vi "Close binary videos refs.vi"(8 "error in":errorcluster, 11 "Cam Binary Videos":refnum<file>[](array[refnum])) -> (0 "error out (no error)":errorcluster)   [LabVIEW 2013]
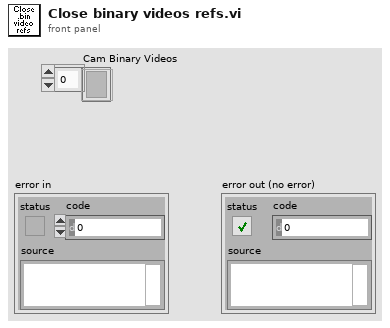
[diagram p1: front panel]
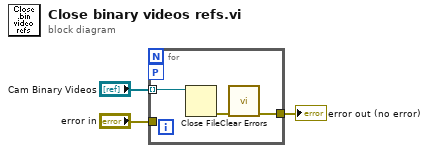
[diagram p0: block diagram]
diagram:
  n1 = for {
    tunnel: "Cam Binary Videos" -> [w5] mode=indexing
    tunnel: "error in" -> [_]
    tunnel: [w4] -> w1
    workers-P: _ -> [_]
    n2 = Close File(refnum=w5) -> (error out=w6:errorcluster)  [unwired: 1 in, 1 out]
    n3 = call <vilib>:"Clear Errors.vi"("error in (no error)"=w6) -> ("error out"=w4:errorcluster)  [unwired: 6 in]
  }
  "error out (no error)" <- w1
